vi "Open Line.vi"(8 "error in (no error)":errorcluster, 9 "Interlock Chain":refnum<class "Interlock Chain.lvclass">, 10 "Sample Line (All Closed)":T1, 11 "Sample Line in":refnum<class "Sample Line.lvclass">) -> (0 "error out":errorcluster, 3 "Sample Line out":refnum<class "Sample Line.lvclass">)   [LabVIEW 2015, in "cRIO-Carbondioxide.lvlib" / "CO2-Actor.lvlib" / "Sample Line.lvclass"]
uses:
  Sample Line.lvclass
  Controls/Sample Line State Enumerator.ctl
  Interlocks/Interlock Chain/Interlock Chain.lvclass
  <vilib>/ActorFramework/Actor/Actor.lvclass/Actor.ctl
  <vilib>/ActorFramework/Message Enqueuer/Message Enqueuer.lvclass/Message Enqueuer.ctl
  Sample Line Messages/Close All Msg/Close All Msg.lvclass/Close All Msg.ctl
  Sample Line.lvclass/Sample Line.ctl
  Valve Messages/Write Bit Field Msg/Write Bit Field Msg.lvclass/Write Bit Field Msg.ctl
  CO2 Actor Messages/Wait Msg/Wait Msg.lvclass/Wait Msg.ctl
  Sample Line Messages/Set Line Status Msg/Set Line Status Msg.lvclass/Set Line Status Msg.ctl
  <vilib>/ActorFramework/Actor/Read Self Enqueuer.vi
  <vilib>/ActorFramework/Message Enqueuer/Enqueue.vi
  <vilib>/ActorFramework/Message Enqueuer/Init from Existing Queue.vi
  <vilib>/ActorFramework/Message Priority Queue/Priority Enqueue.vi
  <vilib>/ActorFramework/Actor/Actor.lvclass
  <vilib>/ActorFramework/Message Enqueuer/Message Enqueuer.lvclass
  Sample Line Messages/Close All Msg/Close All Msg.lvclass
  Valve Messages/Write Bit Field Msg/Write Bit Field Msg.lvclass
  CO2 Actor Messages/Wait Msg/Wait Msg.lvclass
  Sample Line Messages/Set Line Status Msg/Set Line Status Msg.lvclass
  CO2 Actor/CO2 Actor.lvclass
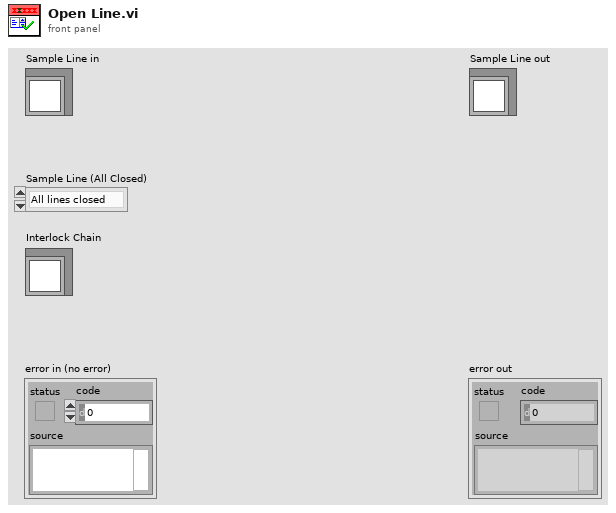
[diagram p1: front panel]
types:
  T1 = typedef "Sample Line State Enumerator.ctl" = enum16{"All lines closed", "Sample line 1.", "Sample line 2.", "Sample line 3.", "Sample line 4.", "Sample line 5.", "Out of range"}
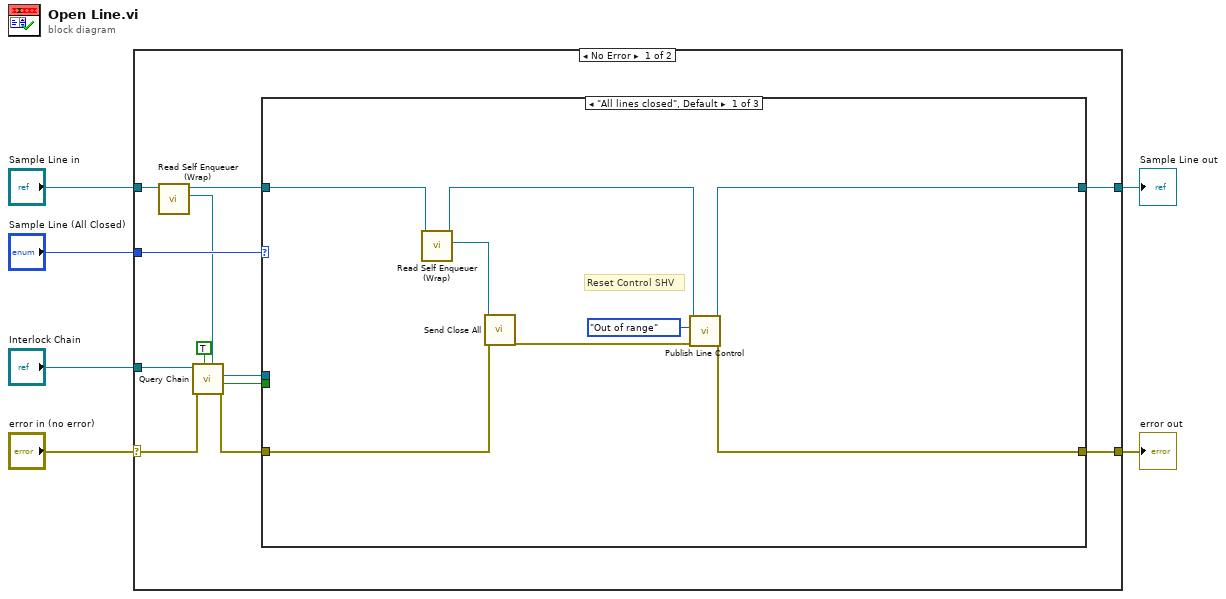
[diagram p0: block diagram]
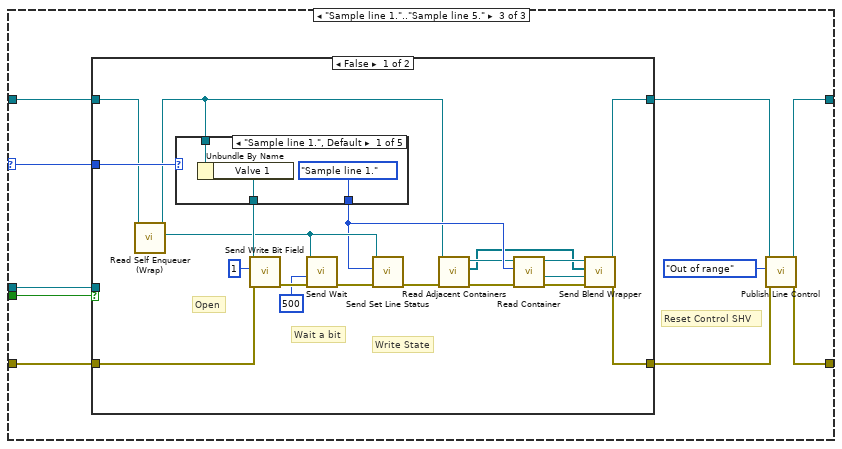
[diagram p3: hidden frame]
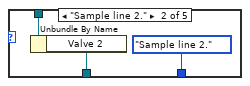
[diagram p4: hidden frame]
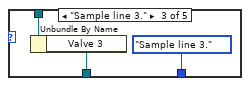
[diagram p5: hidden frame]
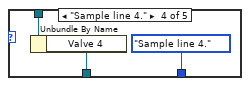
[diagram p6: hidden frame]
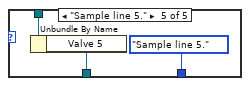
[diagram p7: hidden frame]
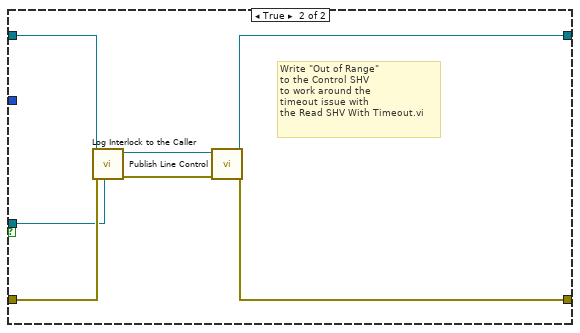
[diagram p8: hidden frame]
diagram:
  n1 = case shown="No Error" "error in (no error)" {
    selector: "error in (no error)" -> [w14 w82]
    tunnel: [w11 w82] -> w5
    tunnel: [w10 w81] -> w3
    tunnel: "Sample Line in" -> [w9 w81]
    tunnel: "Sample Line (All Closed)" -> [w18 _]
    tunnel: "Interlock Chain" -> [w17 _]
    frame No Error {
      n2 = call "Read Self Enqueuer (Wrap).vi"("CO2 Actor in"=w9) -> ("Actor Framework:Message Enqueuer"=w7:refnum<class "Message Enqueuer.lvclass">, "CO2 Actor out"=w8:refnum<class "Sample Line.lvclass">)  [unwired: 9 in]
      n3 = call "Query Chain.vi"("Caller Enqueuer"=w7, "Close Connections (F)"=TRUE ("Close Connections if No Interlock (F)"), "error in (no error)"=w14, "Interlock Chain"=w17) -> ("error out"=w13:errorcluster, "Interlock?"=w15:bool, "Interlock out"=w16:refnum<class "Interlock.lvclass">)  [unwired: 2 in, 3 out]
      n4 = case shown="\"All lines closed\", Default" w18 {
        selector: w18 -> [_ _ w34]
        tunnel: w8 -> [w26 w28 w38]
        tunnel: w13 -> [w24 w27 w37]
        tunnel: [w21 w27 w33] -> w11
        tunnel: [w19 w28 w31] -> w10
        tunnel: w16 -> [_ _ w36]
        tunnel: w15 -> [_ _ w35]
        frame "All lines closed", Default {
          # "Reset Control SHV"
          n5 = call "Read Self Enqueuer (Wrap).vi"("CO2 Actor in"=w26) -> ("Actor Framework:Message Enqueuer"=w25:refnum<class "Message Enqueuer.lvclass">, "CO2 Actor out"=w20:refnum<class "Sample Line.lvclass">)  [unwired: 9 in]
          n6 = call "Send Close All.vi"("error in (no error)"=w24, "Message Enqueuer"=w25) -> ("error out"=w22:errorcluster)  [unwired: 8 in, 1 out]
          n7 = call "Publish Line Control.vi"("error in (no error)"=w22, "Status (Out Of Range)"=Sample_Line_State_Enumerator."Out of range", "Sample Line in"=w20) -> ("error out"=w21:errorcluster, "Sample Line out"=w19:refnum<class "Sample Line.lvclass">)  [unwired: 7 in]
        }
        frame "Out of range" {
        }
        frame "Sample line 1.".."Sample line 5." {
          # "Reset Control SHV"
          n8 = case shown="False" w35 {
            tunnel: w38 -> [w53 w80]
            tunnel: w37 -> [w43 w79]
            tunnel: w36 -> [_ w78]
            tunnel: [w48 w76] -> w32
            tunnel: [w39 w75] -> w30
            tunnel: w34 -> [w57 _]
            frame False {
              # "Write State"
              # "Open"
              # "Wait a bit"
              n9 = call "Read Self Enqueuer (Wrap).vi"("CO2 Actor in"=w53) -> ("Actor Framework:Message Enqueuer"=w54:refnum<class "Message Enqueuer.lvclass">, "CO2 Actor out"=w45:refnum<class "Sample Line.lvclass">)  [unwired: 9 in]
              n10 = case shown="\"Sample line 1.\", Default" w57 {
                tunnel: w45 -> [w61 w64 w67 w70 w73]
                tunnel: [w60 w63 w66 w69 w72] -> w58
                tunnel: [Sample_Line_State_Enumerator."Sample line 1." ("Status (All Closed)") Sample_Line_State_Enumerator."Sample line 2." ("Status (All Closed)") Sample_Line_State_Enumerator."Sample line 3." ("Status (All Closed)") Sample_Line_State_Enumerator."Sample line 4." ("Status (All Closed)") Sample_Line_State_Enumerator."Sample line 5." ("Status (All Closed)")] -> w52
                frame "Sample line 1.", Default {
                  n11 = Unbundle By Name(w61) -> ("Valve 1"=w60:refnum<class "Message Enqueuer.lvclass">)
                }
                frame "Sample line 2." {
                  n12 = Unbundle By Name(w64) -> ("Valve 2"=w63:refnum<class "Message Enqueuer.lvclass">)
                }
                frame "Sample line 3." {
                  n13 = Unbundle By Name(w67) -> ("Valve 3"=w66:refnum<class "Message Enqueuer.lvclass">)
                }
                frame "Sample line 4." {
                  n14 = Unbundle By Name(w70) -> ("Valve 4"=w69:refnum<class "Message Enqueuer.lvclass">)
                }
                frame "Sample line 5." {
                  n15 = Unbundle By Name(w73) -> ("Valve 5"=w72:refnum<class "Message Enqueuer.lvclass">)
                }
              }
              n16 = call "Send Write Bit Field.vi"("error in (no error)"=w43, "Bit Field"=u16 1, "Message Enqueuer"=w58) -> ("error out"=w56:errorcluster)  [unwired: 5 in, 3 out]
              n17 = call "Send Wait.vi"("error in (no error)"=w56, "milliseconds to wait"=u32 500, "Message Enqueuer"=w54) -> ("error out"=w55:errorcluster)  [unwired: 7 in, 1 out]
              n18 = call "Send Set Line Status.vi"("error in (no error)"=w55, "Status (All Closed)"=w52, "Message Enqueuer"=w54) -> ("error out"=w47:errorcluster)  [unwired: 7 in, 1 out]
              n19 = call "Read Adjacent Containers.vi"("error in (no error)"=w47, "Sample Line in"=w45) -> ("error out"=w46:errorcluster, "Adjacent Containers"=w42:refnum<class "Message Enqueuer.lvclass">[], "Sample Line out"=w44:refnum<class "Sample Line.lvclass">)  [unwired: 7 in]
              n20 = call "Read Container.vi"("error in (no error)"=w46, "Sample Line (All Closed)"=w52, "Sample Line in"=w44) -> ("error out"=w51:errorcluster, "Sample"=w50:refnum<class "Sample.lvclass">, "Sample Line out"=w49:refnum<class "Sample Line.lvclass">)  [unwired: 5 in, 1 out]
              n21 = call-dynamic "Send Blend Wrapper.vi"("error in (no error)"=w51, "Sample to Blend"=w50, "Send to"=w42, "CO2 Actor in"=w49) -> ("error out"=w39:errorcluster, "CO2 Actor out"=w48:refnum<class "Sample Line.lvclass">)  [unwired: 6 in]
            }
            frame True {
              # "Write \"Out of Range\"\nto the Control SHV\nto work around the \ntimeout issue with\nthe Read SHV With Timeout.vi"
              n22 = call-dynamic "Log Interlock to the Caller.vi"("Interlock in"=w78, "error in (no error)"=w79, "CO2 Actor in"=w80) -> ("error out"=w74:errorcluster, "CO2 Actor out"=w77:refnum<class "Sample Line.lvclass">)  [unwired: 7 in]
              n23 = call "Publish Line Control.vi"("error in (no error)"=w74, "Sample Line in"=w77) -> ("error out"=w75:errorcluster, "Sample Line out"=w76:refnum<class "Sample Line.lvclass">)  [unwired: 8 in]
            }
          }
          n24 = call "Publish Line Control.vi"("error in (no error)"=w30, "Status (Out Of Range)"=Sample_Line_State_Enumerator."Out of range", "Sample Line in"=w32) -> ("error out"=w33:errorcluster, "Sample Line out"=w31:refnum<class "Sample Line.lvclass">)  [unwired: 7 in]
        }
      }
    }
    frame Error {
    }
  }
  "error out" <- w5
  "Sample Line out" <- w3
